vi "_emi_GFV Loop Enable.vi"(0 "Loop Index/Numb":u16, 1 "Action(Get Index)":T1=enum."Get index", 7 "Loop enable In(T)":bool=TRUE, 11 "error in (no error)":errorcluster) -> (4 "Index out":u16, 8 "Loop Enable Out":bool, 10 "Size":i32, 15 "error out":errorcluster)   [LabVIEW 2011]
uses:
  _emi_Loop control int action.ctl
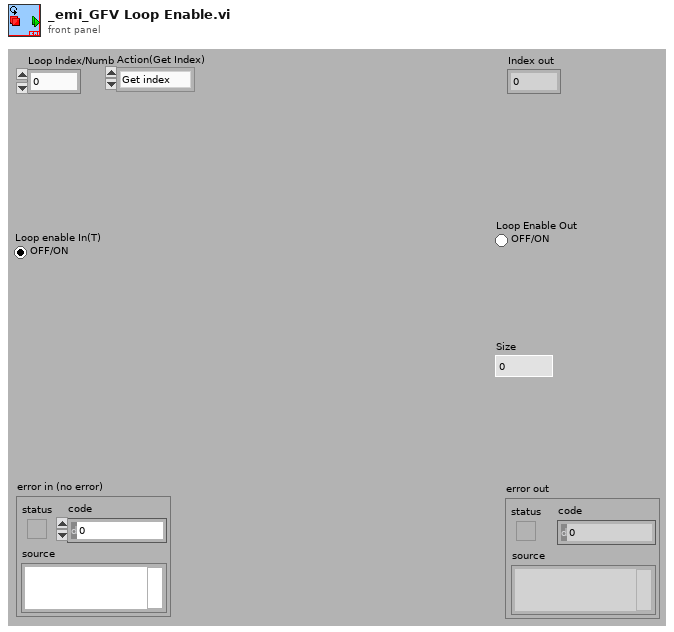
[diagram p1: front panel]
types:
  T1 = typedef "_emi_Loop control int action.ctl" = enum16{"Init index", "Get index", "Set index", "Get Size"}
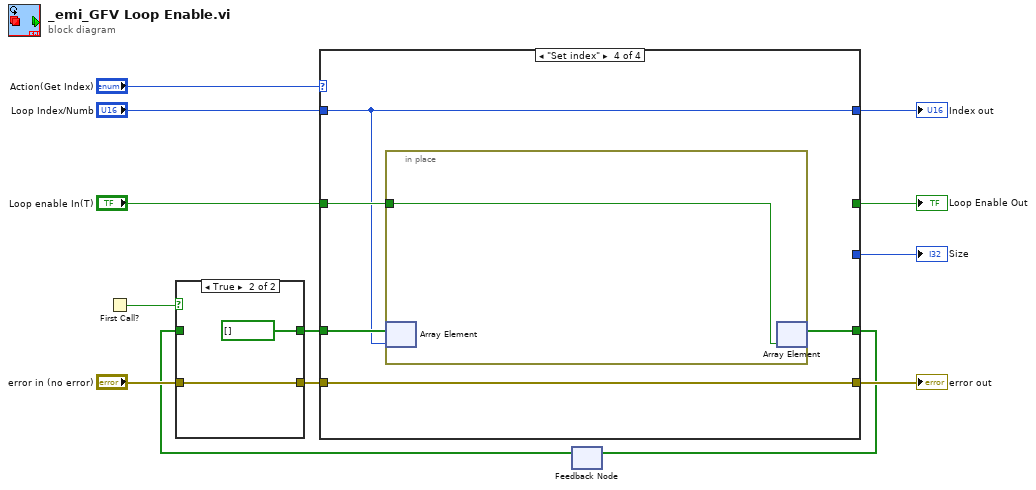
[diagram p0: block diagram]
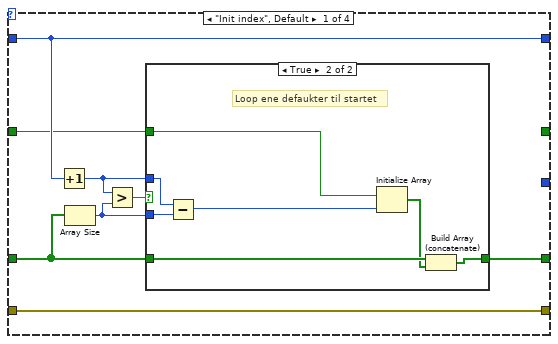
[diagram p2: hidden frame]
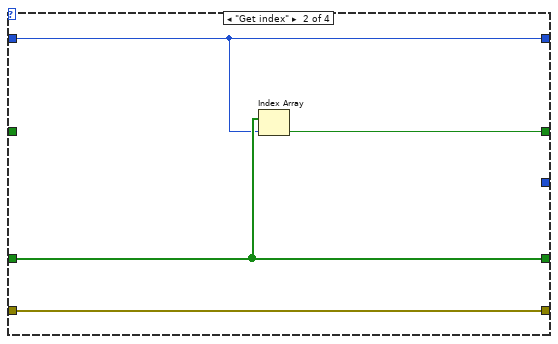
[diagram p4: hidden frame]
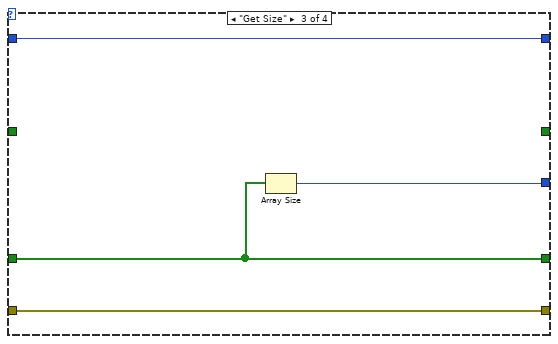
[diagram p5: hidden frame]
diagram:
  n1 = First Call?() -> (First Call?: T/F=w10:bool)
  n2 = feedback #1() -> (w4:bool[])  [unwired: 1 in]
  n3 = case shown="True" w10 {
    tunnel: [w15 w17] -> w12
    tunnel: "error in (no error)" -> [w15 w17]
    tunnel: [w14 bool[] []] -> w5
    tunnel: w4 -> [w14 _]
    frame False {
    }
    frame True {
    }
  }
  n4 = case shown="\"Set index\"" "Action(Get Index)" {
    tunnel: [w25 w37 w41 w46] -> w13
    tunnel: w12 -> [w25 w37 w41 w46]
    tunnel: [w24 w35 w40 w42] -> w9
    tunnel: "Loop Index/Numb" -> [w24 w35 w40 w42]
    tunnel: [w20 w36 w39 w44] -> w6
    tunnel: w5 -> [w19 w36 w39 w45]
    tunnel: [_ w34 _ _] -> w3
    tunnel: "Loop enable In(T)" -> [w18 _ _ w43]
    tunnel: [_ _ w38 _] -> w1
    frame "Init index", Default {
      n5 = Increment(x=w24) -> (x+1=w21:u16)
      n6 = Array Size(array=w19) -> (size(s)=w22:i32)
      n7 = Greater?(x=w21, y=w22) -> (0:w23:bool)
      n8 = case shown="True" w23 {
        tunnel: w22 -> [_ w32]
        tunnel: w21 -> [_ w33]
        tunnel: [w26 w28] -> w20
        tunnel: w19 -> [w26 w30]
        tunnel: w18 -> [_ w27]
        frame False {
        }
        frame True {
          # "Loop ene defaukter til startet"
          n9 = Subtract(x=w33, y=w32) -> (x-y=w31:i32)
          n10 = Initialize Array(w27, w31) -> (w29:bool[])
          n11 = Build Array (concatenate)(w30, w29) -> (w28:bool[])
        }
      }
    }
    frame "Get index" {
      n12 = Index Array(array=w36, index=w35) -> (element=w34:bool)
    }
    frame "Get Size" {
      n13 = Array Size(array=w39) -> (size(s)=w38:i32)
    }
    frame "Set index" {
      n14 = in-place {
        in-place-border: w43 -> [w47]
        n15 = in-place-array #2(w45, w42) -> ()  [unwired: 1 out]
        n16 = in-place-array #2(w47) -> (w44:bool[])  [unwired: 1 out]
      }
    }
  }
  "error out" <- w13
  "Index out" <- w9
  "Loop Enable Out" <- w3
  "Size" <- w1
  n17 = feedback-in #1(w6) -> ()
